vi "_FPGA_DigitalWfm_version2.vi"(9 "Cycle in":u32, 10 "Amplitude*2^29":u32) -> (2 "AuxVoltage":fxp<+/-,16,14>)   [LabVIEW 2018]
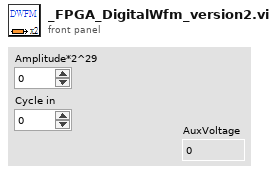
[diagram p1: front panel]
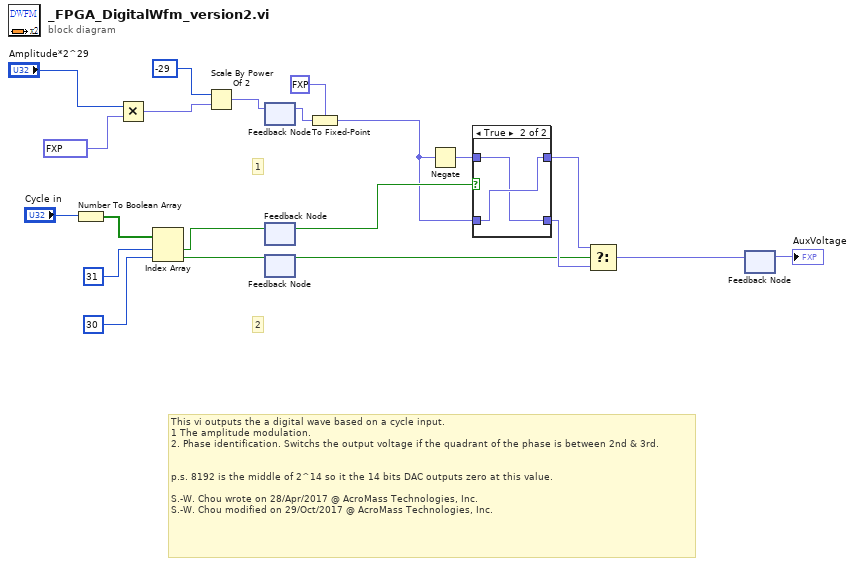
[diagram p0: block diagram]
diagram:
  # "This vi outputs the a digital wave based on a cycle input.\n1 The amplitude modulation.\n2. Phase identification. Switchs the output voltage if the quadrant of the phase is between 2nd & 3rd.\n\n\np.s. 8192 is the middle of 2^14 so it the 14 bits DAC outputs zero at this value.\n\nS.-W. Chou wrote on 28/Apr/2017 @ AcroMass Technologies, Inc.\nS.-W. Chou modified on 29/Oct/2017 @ AcroMass Technologies, Inc."
  # "2"
  # "1"
  n1 = Number To Boolean Array(number="Cycle in") -> (Boolean array=w13:bool[])
  n2 = Multiply(x="Amplitude*2^29", y=fxp<+/-,16,14> 8191.5 ("f")) -> (x*y=w20:fxp<+/-,48,46>)
  n3 = Index Array(array=w13, index #1=31 ("index"), index #2=30 ("index")) -> (element #1=w11:bool, element #2=w9:bool)
  n4 = Scale By Power Of 2(n=i16 -29, x=w20) -> (x*2^n=w17:fxp<+/-,48,46>)
  n5 = feedback #1() -> (w16:fxp<+/-,48,46>)  [unwired: 1 in]
  n6 = feedback-in #1(w17) -> ()
  n7 = feedback-in #2(w11) -> ()
  n8 = feedback #2() -> (w8:bool)  [unwired: 1 in]
  n9 = feedback #3() -> (w5:bool)  [unwired: 1 in]
  n10 = feedback-in #3(w9) -> ()
  n11 = To Fixed-Point(fixed-point type=fxp<+/-,16,14> 0.0 ("cos"), number=w16) -> (fixed-point=w2:fxp<+/-,16,14>)
  n12 = Negate(x=w2) -> (-x=w3:fxp<+/-,17,15>)
  n13 = case shown="True" w8 {
    tunnel: w2 -> [w22 w25]
    tunnel: w3 -> [w23 w24]
    tunnel: [w23 w25] -> w7
    tunnel: [w22 w24] -> w6
    frame False {
    }
    frame True {
    }
  }
  n14 = Select(t=w7, s=w5, f=w6) -> (s? t:f=w1:fxp<+/-,17,15>)
  n15 = feedback #4() -> (→"AuxVoltage":fxp<+/-,17,15>)  [unwired: 1 in]
  n16 = feedback-in #4(w1) -> ()
